vi "SampleAvg.Get Count from BRAM (prefetch).vi"(4 "Step?":bool, 7 "Write Element Data":T1={"Write Index"=0, "Write Element"=0, "Write?"=TRUE}, 8 "Input Valid":bool, 9 "Start New Record":bool) -> (0 "Output Valid":bool, 1 "Start of New Record":bool, 2 "NewCount?":bool, 3 "Next Valid Counts":i16, 6 "Address Pointer":u16)   [LabVIEW 2014]
doc: "<b> Latency = 0 Tick </b>\n<b> Resource Usage : 2 BRAMS of Size 16000 I16 </b>"
panel:
  # "Copyright 2014 Vidrio Technologies\nScanImage 5 software is licensed under the Apache License, Version 2.0 (the \"License\"); you may not use any files contained\nwithin the ScanImage 5 release except in compliance with the License. You may obtain a copy of the License at\n http://www.apache.org/licenses/LICENSE-2.0\nUnless required by applicable law or agreed to in writing, software distributed under the License is distributed on an\n\"AS IS\" BASIS, WITHOUT WARRANTIES OR CONDITIONS OF ANY KIND, either express or implied. See the License for the\n specific language governing permissions and limitations under the License."
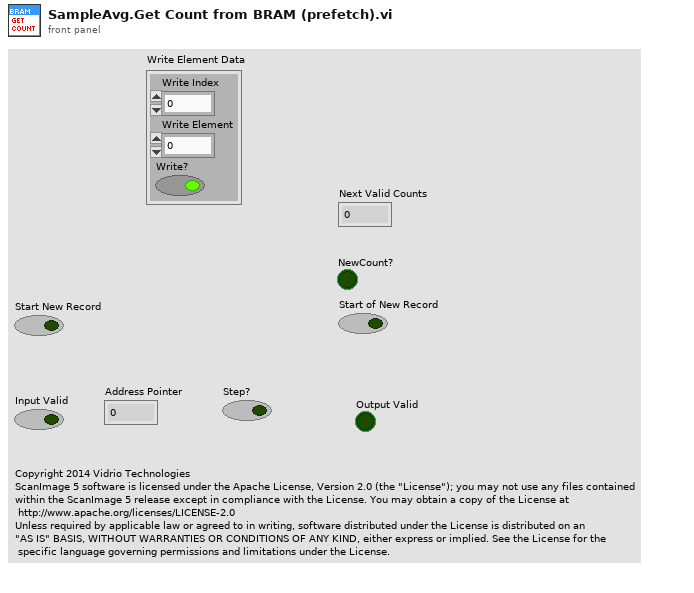
[diagram p1: front panel]
types:
  T1 = cluster{"Write Index":i32, "Write Element":i16, "Write?":bool}
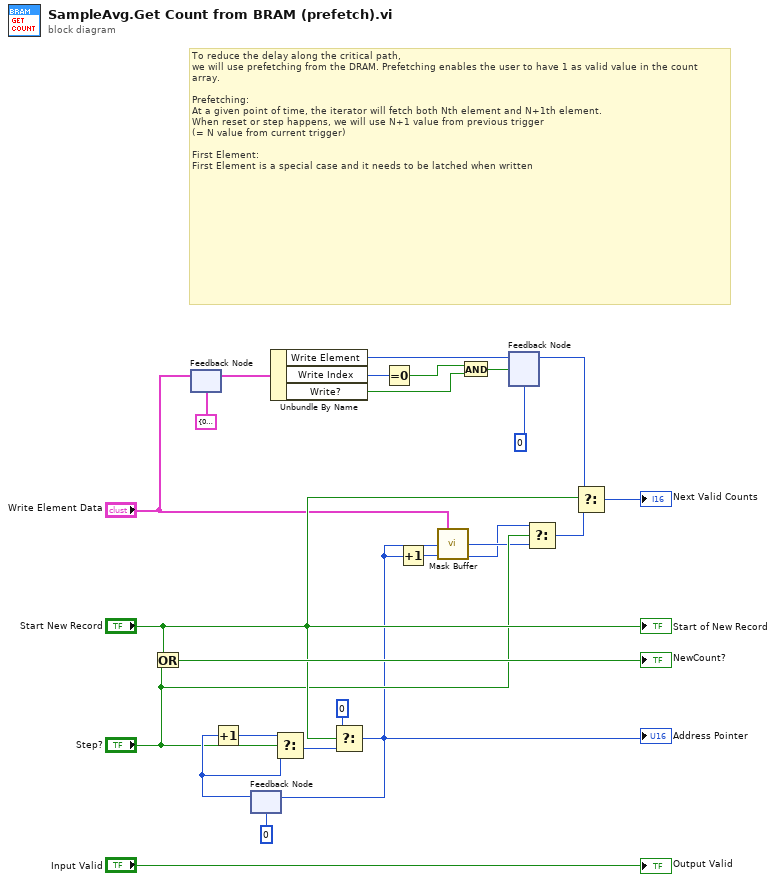
[diagram p0: block diagram]
diagram:
  # "To reduce the delay along the critical path,\nwe will use prefetching from the DRAM. Prefetching enables the user to have 1 as valid value in the count array.\n\nPrefetching:\nAt a given point of time, the iterator will fetch both Nth element and N+1th element.\nWhen reset or step happens, we will use N+1 value from previous trigger \n(= N value from current trigger)\n\nFirst Element:\nFirst Element is a special case and it needs to be latched when written"
  n1 = Or(x="Start New Record", y="Step?") -> (x .or. y?=→"NewCount?":bool)
  n2 = feedback-in #1("Write Element Data") -> ()
  n3 = feedback #1(T1 {"Write Index"=0, "Write Element"=0, "Write?"=FALSE} ("Write Element Data")) -> (w9:T1)
  n4 = feedback #2(u16 0) -> (w23:u16)
  n5 = Increment(x=w23) -> (x+1=w24:u16)
  n6 = Unbundle By Name(w9) -> ("Write Element"=w7:i16, "Write Index"=w8:i32, "Write?"=w4:bool)
  n7 = Select(t=w24, s="Step?", f=w23) -> (s? t:f=w22:u16)
  n8 = Select(t=u16 0, s="Start New Record", f=w22) -> (s? t:f=w13:u16)
  "Address Pointer" <- w13
  n9 = feedback-in #2(w13) -> ()
  n10 = Equal To 0?(x=w8) -> (x = 0?=w3:bool)
  n11 = Increment(x=w13) -> (x+1=w14:u16)
  n12 = call "Mask Buffer.vi"("Write Data"="Write Element Data", "Read Address 0"=w13, "Read Address 1"=w14) -> ("Output 0"=w12:i16, "Output 1"=w11:i16)  [unwired: 11 in]
  n13 = And(x=w3, y=w4) -> (x .and. y?=w2:bool)
  n14 = feedback-in #3(w7, w2) -> ()
  n15 = feedback #3(i16 0 ("Write Element")) -> (w5:i16)
  n16 = Select(t=w11, s="Step?", f=w12) -> (s? t:f=w20:i16)
  n17 = Select(t=w5, s="Start New Record", f=w20) -> (s? t:f=→"Next Valid Counts":i16)
  "Output Valid" <- "Input Valid"
  "Start of New Record" <- "Start New Record"
